vi "UMLEditor Main.vi"(1 "StartProject":string, 3 "StartTarget":string) -> ()   [LabVIEW 2012] (continued)
                                tunnel: w1808 -> [w1870 _ _ _]
                                tunnel: w1799 -> [w1869 _ _ _]
                                tunnel: w1806 -> [_ _ _ _]
                                tunnel: w1798 -> [w1868 _ _ _]
                                frame 0 {
                                n622 = case shown="False" w1870 {
                                tunnel: w1869 -> [_ _]
                                tunnel: w1868 -> [_ w1874]
                                frame False {
                                }
                                frame True {
                                n623 = call <resource>:"GDSProject_GetProjects.vi"("OpenProjectRef(True)"=FALSE) -> ("Projects"=w1877:string[], "error out"=w1880:errorcluster)  [unwired: 2 in, 15 out]
                                n624 = Array Size(array=w1877) -> (size(s)=w1876:i32)
                                n625 = Empty Array?(array=w1877) -> (empty?=w1881:bool)
                                n626 = Decrement(x=w1876) -> (x-1=w1875:i32)
                                n627 = Max & Min(x=w1875, y=w1874) -> (min(x,y)=w1873:i32)  [unwired: 1 out]
                                n628 = Max & Min(x=w1873, y=0) -> (max(x,y)=w1871:i32)  [unwired: 1 out]
                                n629 = Index Array(array=w1877, index=w1871) -> (element=w1879:string)
                                n630 = property on="Project" class="Ring (strict)"("Strings []"=w1877, "Value"=w1871) -> ()  [unwired: 2 in, 2 out]
                                n631 = case shown="False" w1881 {
                                tunnel: w1879 -> [w1887 _]
                                tunnel: w1880 -> [w1888 w1898]
                                tunnel: [w1885 w1897] -> _
                                frame False {
                                n632 = call <resource>:"GetRelativePathOption.vi"() -> ("UseProjectFolderAsBasePath"=w1890:bool)  [unwired: 1 in, 18 out]
                                n633 = call <resource>:"UMLEditor_TargetDialog.vi"("error in (no error)"=w1888, "Target"="My Computer" ("element"), "GetProjectRefByName"=w1887) -> ("error out"=w1885:errorcluster, "ProjectFolder"=w1886:path, "TargetIndex"=w1883:u16, "Targets"=w1884:string[])  [unwired: 4 in, 1 out]
                                n634 = case shown="True" w1890 {
                                tunnel: w1886 -> [_ w1892]
                                tunnel: File_StoredPathesActions."Set Path" ("Method (Get Path)") -> [_ w1891]
                                frame False {
                                }
                                frame True {
                                n635 = call <resource>:"File_ApplicationPaths.vi"("PathName"=UMLEditor_StoredPathes."ClassBasePath" ("UMLPathes"), "Path In"=w1892, "Method (Get Path)"=w1891) -> ()  [unwired: 1 in, 16 out]
                                }
                                }
                                n636 = property on="Target" class="Ring (strict)"("Strings []"=w1884, "Value"=w1883) -> ()  [unwired: 2 in, 2 out]
                                }
                                frame True {
                                n637 = call <resource>:"CommonVIs_UmlOpenVIRef.vi"("ProjectNameIn"="clear", "error in"=w1898) -> ("error out"=w1897:errorcluster)  [unwired: 2 in, 7 out]
                                n638 = property on="Target" class="Ring (strict)"("Strings []"=string[] [], "Value"=u16 0 ("icon")) -> ()  [unwired: 2 in, 2 out]
                                }
                                }
                                }
                                }
                                }
                                frame 1 {
                                }
                                frame 2 {
                                }
                                frame Default {
                                }
                                }
                                n639 = case shown="False" w1812 {
                                tunnel: w1814 -> [w1864 w1867]
                                tunnel: [w1864 w1866] -> w1813
                                frame False {
                                }
                                frame True {
                                n640 = Bundle By Name(cluster=w1867, "state"=UMLEditor_statesType."AddNodeFromProjectTree") -> (w1866:T7)
                                }
                                }
                              }
                              frame True {
                                n641 = Unbundle By Name(w1908) -> ("Cursors"=w1911:refnum<k1>[])
                                n642 = case shown="\"Expand\", \"Collaps\"" w1905 {
                                tunnel: w1911 -> [w1917 _]
                                tunnel: w1910 -> [w1913 w1923]
                                tunnel: [w1913 w1923] -> w1909
                                tunnel: w1905 -> [w1915 _]
                                tunnel: w1903 -> [w1912 w1922]
                                frame Default {
                                n643 = case shown="\"N\", \"S\"" w1915 {
                                tunnel: [_ UMLEditor_Cursortype."NS" ("CursorType") UMLEditor_Cursortype."NESW" ("CursorType") UMLEditor_Cursortype."WE" ("CursorType") UMLEditor_Cursortype."NWSE" ("CursorType")] -> w1914
                                frame Default {
                                }
                                frame "N", "S" {
                                }
                                frame "NE", "SW" {
                                }
                                frame "E", "W" {
                                }
                                frame "SE", "NW" {
                                }
                                }
                                n644 = Index Array(array=w1917, index=w1914) -> (element=w1916:refnum<k1>)
                                n645 = call-poly <vilib>:"Set Cursor.vi"("error in (no error)"=w1913, "VI reference (current VI)"=w1912, "cursor ID"=w1916) -> ()  [unwired: 9 out]
                                }
                                frame "Expand", "Collaps" {
                                n646 = call-poly <vilib>:"Set Cursor.vi"("error in (no error)"=w1923, "VI reference (current VI)"=w1922, "icon"=u16 6) -> ()  [unwired: 9 out]
                                }
                                }
                                n647 = Bundle By Name(cluster=w1907, "HotSpotNode"=w1904) -> (w1906:T7)
                              }
                            }
                          }
                          frame True {
                            n648 = property class="VI"() -> ("Front Panel.IsFrontmost"=w1926:bool)  [unwired: 2 in, 2 out]
                            n649 = case shown="True" w1926 {
                              tunnel: w1925 -> [_ w1945]
                              tunnel: w1934 -> [_ w1944]
                              tunnel: w1933 -> [_ w1943]
                              tunnel: w1932 -> [w1936 w1942]
                              tunnel: [w1936 w1941] -> w1931
                              tunnel: [w1935 w1940] -> w1930
                              tunnel: w1929 -> [w1935 w1939]
                              tunnel: w1928 -> [_ w1938]
                              tunnel: w1927 -> [_ w1937]
                              frame False {
                              }
                              frame True {
                                n650 = case shown="True" w1943 {
                                tunnel: w1945 -> [w1946 w1981]
                                tunnel: w1944 -> [w1974 _]
                                tunnel: w1942 -> [w1956 w1984]
                                tunnel: [w1956 w1985] -> w1941
                                tunnel: [w1968 w1983] -> w1940
                                tunnel: w1939 -> [w1968 w1982]
                                tunnel: w1938 -> [w1952 _]
                                tunnel: w1937 -> [_ _]
                                frame False {
                                w1960 = 0 ("lower limit")
                                n651 = Unbundle By Name(w1956) -> ("zoom"=w1953:dbl)
                                n652 = Multiply(x=w1953, y=w1974) -> (x*y=w1955:dbl)
                                n653 = Multiply(x=w1953, y=w1952) -> (x*y=w1954:dbl)
                                n654 = In Range and Coerce(upper limit=10, x=w1946, lower limit=-10) -> ()  [unwired: 2 out]
                                n655 = property on="Picture" class="Pict"() -> ("Draw Area Size"=w1977:T43)  [unwired: 2 in, 2 out]
                                n656 = To Long Integer(number=w1954) -> (32bit integer=w1964:i32)
                                n657 = To Long Integer(number=w1955) -> (32bit integer=w1971:i32)
                                n658 = property on="Picture" class="Pict"() -> ("Origin:Top"=w1950:i16, "Origin:Left"=w1959:i16)  [unwired: 2 in, 2 out]
                                n659 = Unbundle By Name(w1977) -> ("Height"=w1973:u32, "Width"=w1965:u32)
                                n660 = Subtract(x=w1950, y=w1946) -> (x-y=w1976:i32)
                                n661 = Subtract(x=w1959, y=w1946) -> (x-y=w1958:i32)
                                n662 = To Long Integer(number=w1965) -> (32bit integer=w1963:i32)
                                n663 = Subtract(x=w1964, y=w1963) -> (x-y=w1962:i32)
                                n664 = Max & Min(x=w1962, y=w1960) -> (max(x,y)=w1961:i32)  [unwired: 1 out]
                                n665 = In Range and Coerce(upper limit=w1961, x=w1958, lower limit=w1960) -> (coerced(x)=w1957:i32)  [unwired: 1 out]
                                n666 = To Long Integer(number=w1973) -> (32bit integer=w1966:i32)
                                n667 = Subtract(x=w1971, y=w1966) -> (x-y=w1972:i32)
                                n668 = Max & Min(x=w1972, y=0 ("lower limit")) -> (max(x,y)=w1969:i32)  [unwired: 1 out]
                                n669 = In Range and Coerce(upper limit=w1969, x=w1976, lower limit=0) -> (coerced(x)=w1951:i32)  [unwired: 1 out]
                                n670 = Not Equal?(x=w1951, y=w1950) -> (x != y?=w1949:bool)
                                n671 = Select(t=w1959, s=w1949, f=w1957) -> (s? t:f=w1967:i32)
                                n672 = property on="Picture" class="Pict"("Origin:Top"=w1951, "Origin:Left"=w1967) -> ()  [unwired: 2 in, 2 out]
                                }
                                frame True {
                                w1986 = 1.5 ("x")
                                n673 = Unbundle By Name(w1984) -> ("graphics"=w1993:refnum<class "Graphics.lvclass">, "zoom"=w1979:dbl)
                                n674 = Less Than 0?(x=w1981) -> (x < 0?=w1991:bool)
                                n675 = Not(x=w1991) -> (.not. x?=w1978:bool)
                                n676 = Multiply(x=w1979, y=w1986) -> (x*y=w1992:dbl)
                                n677 = Divide(x=w1979, y=w1986) -> (x/y=w1990:dbl)
                                n678 = Select(t=w1992, s=w1978, f=w1990) -> (s? t:f=w1989:dbl)
                                n679 = In Range and Coerce(upper limit=5.0625, x=w1989, lower limit=0.197530864) -> (coerced(x)=w1980:dbl)  [unwired: 1 out]
                                n680 = call <resource>:"scale.vi"("reference"=w1993, "scaleX"=w1980, "scaleY"=w1980, "error in (no error)"=w1982) -> ("error out"=w1983:errorcluster)  [unwired: 15 out]
                                n681 = Bundle By Name(cluster=w1984, "zoom"=w1980, "state"=UMLEditor_statesType."Repaint") -> (w1985:T7)
                                }
                                }
                              }
                            }
                          }
                        }
                        n682 = Bundle By Name(cluster=w1756, "HotSpotCursor"=w1754, "HotSpotFunction"=w1753) -> (w1755:T7)
                      }
                      frame True {
                        n683 = disable-structure shown="Disabled" {
                          frame Disabled {
                            n684 = property class="VI"() -> ("Front Panel Window:Panel Bounds"=w2011:T53)  [unwired: 2 in, 2 out]
                            n685 = Unbundle By Name(w2011) -> ("Left"=w2005:i16, "Top"=w2002:i16, "Right"=w2006:i16, "Bottom"=w2003:i16)
                            n686 = Subtract(x=w2003, y=w2002) -> (x-y=w2001:i16)
                            n687 = Subtract(x=w2006, y=w2005) -> (x-y=w2004:i16)
                            n688 = Subtract(x=w2004, y=23 ("X")) -> (x-y=w2010:i32)
                            n689 = Subtract(x=w2001, y=100) -> (x-y=w2009:i32)
                            n690 = Bundle(w2010, w2009) -> (w2000:cluster{i32, i32})  [unwired: 1 in]
                            n691 = property on="Picture" class="Pict"("Draw Area Size"=w2000) -> ()  [unwired: 2 in, 2 out]
                          }
                          frame Enabled {
                          }
                        }
                        n692 = Bundle By Name(cluster=w1999, "state"=UMLEditor_statesType."Repaint", "ResizePanelInProgress"=FALSE) -> (w1997:T7)
                      }
                    }
                  }
                  frame True {
                    n693 = property on="Picture" class="Pict"() -> ("Mouse"=w2016:T42)  [unwired: 2 in, 2 out]
                    n694 = Unbundle By Name(w2016) -> ("Mouse Position"=w2015:cluster{"X":i32, "Y":i32})
                    n695 = Unbundle By Name(w2014) -> ("zoom"=w2023:dbl, "offset"=w2021:T12)
                    n696 = Add(x=w2021, y=w2015) -> (x+y=w2022:T12)
                    n697 = Divide(x=w2022, y=w2023) -> (x/y=w2019:T12)
                    n698 = call-dynamic "findNode.vi"("reference"=w2012, "point2D"=w2019, "error in (no error)"=w2013) -> ("node"=w2020:refnum<class "AbstractNode.lvclass">, "found"=w2017:bool, "error out"=w2018:errorcluster)  [unwired: 13 in, 1 out]
                    n699 = case shown="True" w2017 {
                      tunnel: [w2025 w2028] -> w2024
                      tunnel: w2020 -> [_ w2032]
                      tunnel: w2019 -> [_ w2031]
                      tunnel: w2018 -> [w2025 w2030]
                      frame False {
                      }
                      frame True {
                        n700 = call-dynamic "GetContextHelpInfo.vi"("reference"=w2032, "MousePos"=w2031, "error in (no error)"=w2030) -> ("ContextHelpInfoExist"=w2026:bool, "ContextHelpInfo"=w2027:variant, "error out"=w2029:errorcluster)  [unwired: 13 in, 1 out]
                        n701 = case shown="True" w2026 {
                          tunnel: w2029 -> [w2033 w2036]
                          tunnel: [w2033 w2035] -> w2028
                          tunnel: w2027 -> [_ w2034]
                          frame False {
                          }
                          frame True {
                            n702 = call <resource>:"ContextHelp_SendMessageToPopUp.vi"("PopUpMessage"=w2034, "error in (no error)"=w2036) -> ("error out"=w2035:errorcluster)  [unwired: 1 in, 16 out]
                          }
                        }
                      }
                    }
                  }
                }
              }
              frame True {
                (unwired) UMLEditor_HotSpotType."Expand" ("HotSpotFunction")
                n703 = property on="Picture" class="Pict"() -> ("Mouse"=w2040:T42)  [unwired: 2 in, 2 out]
                n704 = Unbundle By Name(w2040) -> ("Mouse Position.X"=w2069:i32, "Mouse Position.Y"=w2068:i32, "Mouse Position"=w2051:cluster{"X":i32, "Y":i32})
                n705 = Unbundle By Name(w2039) -> ("graphics"=w2065:refnum<class "Graphics.lvclass">, "rubberBandStart"=w2064:T12, "dragStartPoint"=w2048:T12, "dragStartBounds"=w2056:T13, "selcted"=w2047:T9, "lastMousePoint"=w2046:T12)
                n706 = Unbundle By Name(w2039) -> ("HotSpotCursor"=w2042:bool, "HotSpotFunction"=w2044:T19)
                n707 = Unbundle By Name(w2039) -> ("ShiftDown"=w2038:bool, "CtrlDown"=w2037:bool)
                n708 = Unbundle By Name(w2039) -> ("selcted"=w2058:T9, "SelectedNodes"=w2057:refnum<class "AbstractNode.lvclass">[], "selectedEdge"=w2049:refnum<class "AbstractEdge.lvclass">)
                n709 = Unbundle By Name(w2039) -> ("offset"=w2050:T12, "zoom"=w2061:dbl)
                n710 = Add(x=w2051, y=w2050) -> (x+y=w2052:T12)
                n711 = Add(x=w2069, y=w2068) -> (x+y=w2067:i32)
                n712 = Divide(x=w2052, y=w2061) -> (x/y=w2053:T12)
                n713 = Equal?(x=w2046, y=w2053) -> (x = y?=w2054:bool)
                n714 = call <resource>:"Point getValues.vi"("point2D"=w2064) -> ("valid"=w2063:bool)  [unwired: 18 out]
                n715 = call <resource>:"Point getValues.vi"("point2D"=w2048) -> ("valid"=w2062:bool)  [unwired: 18 out]
                n716 = Less Than 0?(x=w2067) -> (x < 0?=w2055:bool)
                n717 = Or(x=w2054, y=w2055) -> (x .or. y?=w2043:bool)
                n718 = Compound Arithmetic op=AND(w2043, invert w2042) -> (w2041:bool)
                n719 = case shown="True" w2041 {
                  tunnel: w2053 -> [w2091 _]
                  tunnel: w2065 -> [w2090 _]
                  tunnel: w2039 -> [w2078 w2314]
                  tunnel: [w2077 w2313] -> w2066
                  tunnel: w2064 -> [w2089 _]
                  tunnel: w2063 -> [w2088 _]
                  tunnel: w2062 -> [w2087 _]
                  tunnel: w2059 -> [w2086 w2312]
                  tunnel: [w2085 w2312] -> w2060
                  tunnel: w2039 -> [w2084 _]
                  tunnel: w2058 -> [w2083 _]
                  tunnel: w2057 -> [w2082 _]
                  tunnel: w2056 -> [w2081 _]
                  tunnel: w2048 -> [w2080 _]
                  tunnel: w2045 -> [w2079 _]
                  tunnel: w2054 -> [_ w2311]
                  tunnel: w2049 -> [w2076 _]
                  tunnel: w2047 -> [w2075 _]
                  tunnel: w2046 -> [w2074 _]
                  tunnel: w2045 -> [w2073 _]
                  tunnel: w2042 -> [w2072 _]
                  tunnel: w2044 -> [w2071 _]
                  tunnel: w2038 -> [_ _]
                  tunnel: w2037 -> [_ _]
                  tunnel: w2037 -> [w2070 _]
                  frame False {
                    n720 = case shown="False" w2088 {
                      tunnel: w2091 -> [w2102 w2279]
                      tunnel: w2090 -> [_ w2286]
                      tunnel: w2089 -> [_ w2280]
                      tunnel: w2087 -> [w2109 _]
                      tunnel: w2086 -> [w2107 w2285]
                      tunnel: [w2108 w2284] -> w2085
                      tunnel: w2084 -> [w2106 _]
                      tunnel: w2083 -> [w2105 _]
                      tunnel: w2082 -> [w2104 _]
                      tunnel: w2081 -> [w2103 _]
                      tunnel: w2080 -> [w2101 _]
                      tunnel: w2079 -> [w2100 _]
                      tunnel: w2078 -> [w2099 w2283]
                      tunnel: [w2098 w2282] -> w2077
                      tunnel: w2076 -> [w2097 _]
                      tunnel: w2075 -> [_ w2281]
                      tunnel: w2074 -> [w2096 _]
                      tunnel: w2073 -> [w2095 _]
                      tunnel: w2072 -> [w2094 _]
                      tunnel: w2071 -> [w2093 _]
                      tunnel: w2070 -> [w2092 _]
                      frame False {
                        n721 = case shown="True" w2109 {
                          tunnel: [w2111 w2125] -> w2108
                          tunnel: w2107 -> [w2111 w2126]
                          tunnel: w2106 -> [_ _]
                          tunnel: w2105 -> [_ w2127]
                          tunnel: w2104 -> [_ w2124]
                          tunnel: w2103 -> [_ w2117]
                          tunnel: w2102 -> [_ w2123]
                          tunnel: w2101 -> [_ w2122]
                          tunnel: w2100 -> [_ w2121]
                          tunnel: w2099 -> [w2110 w2120]
                          tunnel: [w2110 w2119] -> w2098
                          tunnel: w2097 -> [_ w2118]
                          tunnel: w2096 -> [_ w2116]
                          tunnel: w2095 -> [_ w2115]
                          tunnel: w2094 -> [_ w2114]
                          tunnel: w2093 -> [_ w2113]
                          tunnel: w2092 -> [_ w2112]
                          frame False {
                          }
                          frame True {
                            n722 = case shown="\"Edge\"" w2127 {
                              tunnel: w2126 -> [w2129 w2136 w2256]
                              tunnel: [w2129 w2140 w2264] -> w2125
                              tunnel: w2124 -> [_ w2134 w2255]
                              tunnel: w2123 -> [_ w2137 w2254]
                              tunnel: w2122 -> [_ _ w2270]
                              tunnel: w2121 -> [_ _ w2267]
                              tunnel: w2120 -> [w2128 w2142 w2266]
                              tunnel: [w2128 w2138 w2262] -> w2119
                              tunnel: w2118 -> [_ _ w2261]
                              tunnel: w2117 -> [_ _ _]
                              tunnel: w2116 -> [_ w2135 _]
                              tunnel: w2115 -> [_ w2133 _]
                              tunnel: w2114 -> [_ w2132 _]
                              tunnel: w2113 -> [_ w2131 _]
                              tunnel: w2112 -> [_ w2130 _]
                              frame Default {
                              }
                              frame "Node" {
                                n723 = Bundle By Name(cluster=w2142, "state"=UMLEditor_statesType."Repaint", "lastMousePoint"=w2137) -> (w2139:T7)
                                n724 = case shown="True" w2132 {
                                tunnel: [w2150 w2206] -> w2140
                                tunnel: w2139 -> [w2149 w2202]
                                tunnel: [w2148 w2201] -> w2138
                                tunnel: w2137 -> [w2147 w2210]
                                tunnel: w2136 -> [w2146 w2207]
                                tunnel: w2135 -> [w2145 w2209]
                                tunnel: w2134 -> [w2144 w2205]
                                tunnel: w2133 -> [_ _]
                                tunnel: w2131 -> [_ w2208]
                                tunnel: w2130 -> [w2143 _]
                                frame False {
                                n725 = case shown="False" w2143 {
                                tunnel: [w2160 w2196] -> w2150
                                tunnel: w2149 -> [w2159 w2200]
                                tunnel: [w2158 w2197] -> w2148
                                tunnel: w2147 -> [w2157 _]
                                tunnel: w2146 -> [w2156 w2196]
                                tunnel: w2145 -> [w2155 _]
                                tunnel: w2144 -> [w2154 _]
                                frame False {
                                n726 = for {
                                tunnel: w2154 -> [w2163] mode=indexing
                                shift-right: [w2164] -> w2153
                                shift-left: refnum<class "AbstractNode.lvclass">[] [] -> [w2165]
                                n727 = call <resource>:"GetAllChildrenRecursive.vi"("reference"=w2163) -> ("children"=w2162:refnum<class "AbstractNode.lvclass">[])  [unwired: 1 in, 17 out]
                                n728 = Build Array (concatenate)(w2165, w2162) -> (w2164:refnum<class "AbstractNode.lvclass">[])
                                }
                                n729 = for {
                                tunnel: w2154 -> [w2189] mode=indexing
                                tunnel: w2157 -> [w2185]
                                shift-right: [w2187] -> w2152
                                shift-left: w2156 -> [w2188]
                                tunnel: w2155 -> [w2184]
                                tunnel: w2153 -> [w2171]
                                w2174 = 0.0 ("t")
                                n730 = Subtract(x=w2185, y=w2184) -> (x-y=w2186:T12)
                                n731 = call-dynamic "getBounds.vi"("reference"=w2189, "error in (no error)"=w2188) -> ("reference out"=w2168:refnum<class "AbstractNode.lvclass">, "bounds"=w2183:T13, "error out"=w2169:errorcluster)  [unwired: 15 in]
                                n732 = Unbundle(w2183) -> ("x"=w2182:dbl, "y"=w2176:dbl)  [unwired: 2 out]
                                n733 = Unbundle(w2186) -> ("x"=w2175:dbl, "y"=w2173:dbl)
                                n734 = call-dynamic "getParent.vi"("reference"=w2168, "error in (no error)"=w2169) -> ("reference out"=w2166:refnum<class "AbstractNode.lvclass">, "error out"=w2167:errorcluster)  [unwired: 13 in, 3 out]
                                n735 = Search 1D Array(1D array=w2171, element=w2168) -> (index of element=w2170:i32)  [unwired: 1 out]
                                n736 = Add(x=w2182, y=w2175) -> (x+y=w2181:dbl)
                                n737 = Add(x=w2176, y=w2173) -> (x+y=w2177:dbl)
                                n738 = Less Than 0?(x=w2181) -> (x < 0?=w2180:bool)
                                n739 = Less Than 0?(x=w2177) -> (x < 0?=w2178:bool)
                                n740 = Select(t=w2174, s=w2180, f=w2175) -> (s? t:f=w2179:dbl)
                                n741 = Select(t=w2174, s=w2178, f=w2173) -> (s? t:f=w2172:dbl)
                                n742 = case shown="-1" w2170 {
                                tunnel: w2167 -> [w2190 w2195]
                                tunnel: [w2190 w2194] -> w2187
                                tunnel: w2179 -> [_ w2193]
                                tunnel: w2172 -> [_ w2192]
                                tunnel: w2166 -> [_ w2191]
                                frame 0, Default {
                                }
                                frame -1 {
                                n743 = call-dynamic "translate.vi"("reference"=w2191, "dx"=w2193, "dy"=w2192, "error in (no error)"=w2195) -> ("error out"=w2194:errorcluster)  [unwired: 14 in, 1 out]
                                }
                                }
                                }
                                n744 = call <resource>:"UMLEditor setDiagramInfo.vi"("error in (no error)"=w2152, "localVariablesIn"=w2159, "action"=enum16{"Name/Dir", "Unsaved", "Saved"}."Unsaved") -> ("localVariablesOut"=w2158:T7, "error out"=w2160:errorcluster)  [unwired: 2 in, 13 out]
                                }
                                frame True {
                                n745 = Bundle By Name(cluster=w2200, "state"=UMLEditor_statesType."CopyPaste", "CtrlDown"=FALSE) -> (w2197:T7)
                                }
                                }
                                }
                                frame True {
                                n746 = Subtract(x=w2210, y=w2209) -> (x-y=w2211:T12)
                                n747 = Unbundle(w2211) -> ("x"=w2204:dbl, "y"=w2203:dbl)
                                n748 = case shown="\"Expand\", \"Collaps\"" w2208 {
                                selector: w2208 -> [_ w2219 w2236]
                                tunnel: w2207 -> [w2213 w2218 w2241]
                                tunnel: [w2213 w2216 w2240] -> w2206
                                tunnel: w2205 -> [_ w2217 w2239]
                                tunnel: w2204 -> [_ _ w2238]
                                tunnel: w2203 -> [_ _ w2237]
                                tunnel: w2202 -> [w2212 w2215 w2235]
                                tunnel: [w2212 w2214 w2235] -> w2201
                                frame Default {
                                }
                                frame "Expand", "Collaps" {
                                n749 = disable-structure shown="Disabled" {
                                disable-tunnel: w2219 -> [w2232 _]
                                disable-tunnel: w2218 -> [w2229 w2233]
                                disable-tunnel: w2217 -> [w2228 _]
                                disable-tunnel: [w2224 w2233] -> w2216
                                disable-tunnel: w2215 -> [w2223 w2234]
                                disable-tunnel: [w2220 w2234] -> w2214
                                frame Disabled {
                                n750 = Index Array(array=w2228) -> (element=w2227:refnum<class "AbstractNode.lvclass">)  [unwired: 1 in]
                                n751 = Equal?(x=w2232, y=UMLEditor_HotSpotType."Collaps") -> (x = y?=w2230:bool)
                                n752 = call-dynamic "Collaps.vi"("reference in"=w2227, "Collaps"=w2230, "error in (no error)"=w2229) -> ("error out"=w2225:errorcluster)  [unwired: 15 in, 1 out]
                                n753 = Bundle By Name(cluster=w2223, "HotSpotCursor"=FALSE) -> (w2221:T7)
                                n754 = call <resource>:"UMLEditor setDiagramInfo.vi"("error in (no error)"=w2225, "localVariablesIn"=w2221, "action"=enum16{"Name/Dir", "Unsaved", "Saved"}."Unsaved") -> ("localVariablesOut"=w2220:T7, "error out"=w2224:errorcluster)  [unwired: 2 in, 13 out]
                                }
                                frame Enabled {
                                }
                                }
                                }
                                frame "N".."NW" {
                                n755 = for {
                                shift-right: [w2246] -> w2240
                                shift-left: w2241 -> [w2247]
                                tunnel: w2239 -> [w2245] mode=indexing
                                tunnel: w2238 -> [w2244]
                                tunnel: w2237 -> [w2243]
                                tunnel: w2236 -> [w2242]
                                n756 = call-dynamic "Resize.vi"("reference in"=w2245, "dx"=w2244, "dy"=w2243, "Positions"=w2242, "error in (no error)"=w2247) -> ("error out"=w2246:errorcluster)  [unwired: 13 in, 1 out]
                                }
                                }
                                }
                                }
                                }
                              }
                              frame "Edge" {
                                n757 = Array Size(array=w2255) -> (size(s)=w2248:i32)
                                n758 = Unbundle By Name(w2270) -> ("x"=w2269:dbl, "y"=w2268:dbl)
                                n759 = case shown="2" w2248 {
                                tunnel: w2255 -> [_ w2274]
                                tunnel: [w2272 w2273] -> w2250
                                frame 2 {
                                n760 = call <resource>:"GetObject.vi"("RefNum"=-1 ("type")) -> ("reference"=w2272:refnum<class "AbstractNode.lvclass">)  [unwired: 17 in, 1 out]
                                }
                                frame Default {
                                n761 = Index Array(array=w2274) -> (element=w2273:refnum<class "AbstractNode.lvclass">)  [unwired: 1 in]
                                }
                                }
                                n762 = Unbundle(w2254) -> ("x"=w2258:dbl, "y"=w2257:dbl)
                                n763 = Subtract(x=w2258, y=w2269) -> (x-y=w2260:dbl)
                                n764 = Subtract(x=w2257, y=w2268) -> (x-y=w2259:dbl)
                                n765 = Bundle By Name(cluster=w2266, "state"=UMLEditor_statesType."Repaint", "lastMousePoint"=w2254, "dragStartPoint"=w2254) -> (w2263:T7)
                                n766 = call-dynamic "Translate.vi"("reference"=w2261, "dx"=w2260, "dy"=w2259, "StartEndNode"=w2250, "error in (no error)"=w2256) -> ("error out"=w2251:errorcluster)  [unwired: 13 in, 1 out]
                                n767 = case shown="False" "Case Constant\n(See Context Help) 2" {
                                tunnel: w2267 -> [_ w2278]
                                tunnel: [w2275 w2277] -> w2252
                                tunnel: w2251 -> [w2275 w2276]
                                frame False {
                                }
                                frame True {
                                n768 = call-dynamic "layout.vi"("reference"=w2278, "error in (no error)"=w2276) -> ("error out"=w2277:errorcluster)  [unwired: 16 in, 1 out]
                                }
                                }
                                n769 = call <resource>:"UMLEditor setDiagramInfo.vi"("error in (no error)"=w2252, "localVariablesIn"=w2263, "action"=enum16{"Name/Dir", "Unsaved", "Saved"}."Unsaved") -> ("localVariablesOut"=w2262:T7, "error out"=w2264:errorcluster)  [unwired: 2 in, 13 out]
                              }
                            }
                          }
                        }
                      }
                      frame True {
                        n770 = case shown="\"None\"" w2281 {
                          tunnel: w2286 -> [w2302 w2310]
                          tunnel: w2285 -> [w2304 w2309]
                          tunnel: [w2303 w2308] -> w2284
                          tunnel: w2280 -> [w2297 w2306]
                          tunnel: w2279 -> [w2296 w2305]
                          frame "None" {
                            n771 = Unbundle(w2297) -> ("x"=w2295:dbl, "y"=w2291:dbl)
                            n772 = Unbundle(w2296) -> ("x"=w2294:dbl, "y"=w2290:dbl)
                            n773 = Max & Min(x=w2295, y=w2294) -> (max(x,y)=w2293:dbl, min(x,y)=w2292:dbl)
                            n774 = Max & Min(x=w2291, y=w2290) -> (max(x,y)=w2289:dbl, min(x,y)=w2288:dbl)
                            n775 = Subtract(x=w2293, y=w2292) -> (x-y=w2299:dbl)
                            n776 = Subtract(x=w2289, y=w2288) -> (x-y=w2298:dbl)
                            n777 = Bundle By Name(cluster=T13 {"x"=0.0, "y"=0.0, "width"=0.0, "height"=0.0} ("rectangle"), "x"=w2292, "y"=w2288, "width"=w2299, "height"=w2298) -> (w2287:T13)
                            n778 = call <resource>:"drawTempRectangle.vi"("reference"=w2302, "rectangle"=w2287, "color(if not used=default color)"=u32 16711680, "error in (no error)"=w2304) -> ("error out"=w2303:errorcluster)  [unwired: 4 in, 11 out]
                          }
                          frame Default {
                            n779 = Build Array(w2306, w2305) -> (w2307:T12[])
                            n780 = call-dynamic "drawTempLine.vi"("reference"=w2310, "points"=w2307, "error in (no error)"=w2309) -> ("error out"=w2308:errorcluster)  [unwired: 15 in, 1 out]
                          }
                        }
                        n781 = Bundle By Name(cluster=w2283, "lastMousePoint"=w2279) -> (w2282:T7)
                      }
                    }
                  }
                  frame True {
                    n782 = case shown="True" w2311 {
                      tunnel: w2314 -> [w2318 w2320]
                      tunnel: [w2317 w2320] -> w2313
                      frame False {
                        w2316 = T12 {"x"=nan, "y"=nan} ("rubberBandStart")
                        n783 = Bundle By Name(cluster=w2318, "butDwn"=FALSE ("b_dwn"), "rubberBandStart"=w2316, "dragStartPoint"=w2316, "dragStartBounds"=T13 {"x"=nan, "y"=nan, "width"=nan, "height"=nan}) -> (w2317:T7)
                      }
                      frame True {
                      }
                    }
                  }
                }
              }
            }
          }
          event User Event {
            # "WholeProject"
            # "ReverseEngineering:Class:%s:%s"
            n784 = event-data() -> ("Action"=w2322:string, "Data"=w2321:string)  [unwired: 1 out]
            n785 = case shown="\"ReverseEngineering\"" w2322 {
              tunnel: w2326 -> [w2328 w2352 w2405 w2426]
              tunnel: [w2328 w2351 w2404 w2425] -> w2325
              tunnel: w2321 -> [_ w2350 w2403 w2427]
              tunnel: w2324 -> [w2327 w2348 w2401 w2423]
              tunnel: [w2327 w2347 w2400 w2423] -> w2323
              frame "False", Default {
              }
              frame "ReverseEngineering" {
                n786 = Match Pattern(string=w2350, regular expression=":") -> (before substring=w2337:string, after substring=w2345:string)  [unwired: 3 out]
                n787 = Match Pattern(string=w2345, regular expression=":") -> (before substring=w2344:string, after substring=w2335:string)  [unwired: 3 out]
                n788 = Reverse String(1:w2335) -> (0:w2334:string)
                n789 = Match Pattern(string=w2334, regular expression=":") -> (before substring=w2333:string, after substring=w2332:string)  [unwired: 3 out]
                n790 = Reverse String(1:w2333) -> (0:w2330:string)
                n791 = Reverse String(1:w2332) -> (0:w2331:string)
                n792 = call <resource>:"GDSProject_GetProjects.vi"("error in (no error)"=w2348, "OpenProjectRef(True)"=FALSE) -> ("Projects"=w2340:string[], "error out"=w2342:errorcluster)  [unwired: 1 in, 15 out]
                n793 = case shown="\"WholeProject\"" w2337 {
                  tunnel: w2352 -> [w2356 w2360 w2364]
                  tunnel: [w2355 w2359 w2363] -> w2351
                  tunnel: w2337 -> [w2354 _ _]
                  tunnel: w2331 -> [_ w2357 w2361]
                  frame "WholeProject" {
                    n794 = Bundle By Name(cluster=w2356, "Action"=w2354, "state"=UMLEditor_statesType."ClassReversedEngineering") -> (w2355:T7)
                  }
                  frame Default {
                    n795 = Bundle By Name(cluster=w2360, "Action"=w2357, "state"=UMLEditor_statesType."ClassReversedEngineering") -> (w2359:T7)
                  }
                  frame "VI" {
                    n796 = Bundle By Name(cluster=w2364, "Action"=w2361, "state"=UMLEditor_statesType."AddNodeFromProjectTree+SyncAll") -> (w2363:T7)
                  }
                }
                n797 = Search 1D Array(1D array=w2340, element=w2344) -> (index of element=w2339:i32)  [unwired: 1 out]
                n798 = case shown="0, Default" w2339 {
                  selector: w2339 -> [w2365 _]
                  tunnel: [w2365 0 ("t")] -> w2338
                  frame 0, Default {
                  }
                  frame -1 {
                  }
                }
                n799 = Index Array(array=w2340, index=w2338) -> (element=w2343:string)
                n800 = Empty Array?(array=w2340) -> (empty?=w2341:bool)
                n801 = property on="Project" class="Ring (strict)"("Strings []"=w2340, "Value"=w2338) -> ()  [unwired: 2 in, 2 out]
                n802 = case shown="True" w2341 {
                  tunnel: w2343 -> [w2374 _]
                  tunnel: w2342 -> [w2375 w2381]
                  tunnel: [w2373 w2381] -> w2347
                  tunnel: w2330 -> [w2370 _]
                  frame False {
                    n803 = call <resource>:"UMLEditor_TargetDialog.vi"("error in (no error)"=w2375, "Target"=w2370, "GetProjectRefByName"=w2374) -> ("error out"=w2373:errorcluster, "ProjectFolder"=w2367:path, "TargetIndex"=w2371:u16, "Targets"=w2372:string[])  [unwired: 4 in, 1 out]
                    n804 = call <resource>:"GetRelativePathOption.vi"() -> ("UseProjectFolderAsBasePath"=w2369:bool)  [unwired: 1 in, 18 out]
                    n805 = case shown="True" w2369 {
                      tunnel: w2367 -> [_ w2377]
                      tunnel: File_StoredPathesActions."Set Path" ("Method (Get Path)") -> [_ w2376]
                      frame False {
                      }
                      frame True {
                        n806 = call <resource>:"File_ApplicationPaths.vi"("PathName"=UMLEditor_StoredPathes."ClassBasePath" ("UMLPathes"), "Path In"=w2377, "Method (Get Path)"=w2376) -> ()  [unwired: 1 in, 16 out]
                      }
                    }
                    n807 = property on="Target" class="Ring (strict)"("Strings []"=w2372, "Value"=w2371) -> ()  [unwired: 2 in, 2 out]
                  }
                  frame True {
                    n808 = property on="Target" class="Ring (strict)"("Strings []"=string[] [], "Value"=u16 0 ("icon")) -> ()  [unwired: 2 in, 2 out]
                  }
                }
              }
              frame "ShowInStateDiagram" {
                n809 = Match Pattern(string=w2403, regular expression=":") -> (after substring=w2398:string)  [unwired: 4 out]
                n810 = Match Pattern(string=w2398, regular expression=":") -> (before substring=w2397:string, after substring=w2383:string)  [unwired: 3 out]
                n811 = Reverse String(1:w2383) -> (0:w2388:string)
                n812 = Match Pattern(string=w2388, regular expression=":") -> (before substring=w2387:string, after substring=w2386:string)  [unwired: 3 out]
                n813 = Reverse String(1:w2387) -> (0:w2384:string)
                n814 = Reverse String(1:w2386) -> (0:w2385:string)
                n815 = call <resource>:"GDSProject_GetProjects.vi"("error in (no error)"=w2401, "OpenProjectRef(True)"=FALSE) -> ("Projects"=w2393:string[], "error out"=w2395:errorcluster)  [unwired: 1 in, 15 out]
                n816 = Search 1D Array(1D array=w2393, element=w2397) -> (index of element=w2392:i32)  [unwired: 1 out]
                n817 = case shown="-1" w2392 {
                  selector: w2392 -> [w2406 _]
                  tunnel: [w2406 0 ("t")] -> w2391
                  frame 0, Default {
                  }
                  frame -1 {
                  }
                }
                n818 = Index Array(array=w2393, index=w2391) -> (element=w2396:string)
                n819 = Empty Array?(array=w2393) -> (empty?=w2394:bool)
                n820 = property on="Project" class="Ring (strict)"("Strings []"=w2393, "Value"=w2391) -> ()  [unwired: 2 in, 2 out]
                n821 = case shown="True" w2394 {
                  tunnel: w2396 -> [w2415 _]
                  tunnel: w2395 -> [w2416 w2422]
                  tunnel: [w2414 w2422] -> w2400
                  tunnel: w2384 -> [w2411 _]
                  frame False {
                    n822 = call <resource>:"UMLEditor_TargetDialog.vi"("error in (no error)"=w2416, "Target"=w2411, "GetProjectRefByName"=w2415) -> ("error out"=w2414:errorcluster, "ProjectFolder"=w2408:path, "TargetIndex"=w2412:u16, "Targets"=w2413:string[])  [unwired: 4 in, 1 out]
                    n823 = call <resource>:"GetRelativePathOption.vi"() -> ("UseProjectFolderAsBasePath"=w2410:bool)  [unwired: 1 in, 18 out]
                    n824 = property on="Target" class="Ring (strict)"("Strings []"=w2413, "Value"=w2412) -> ()  [unwired: 2 in, 2 out]
                    n825 = case shown="True" w2410 {
                      tunnel: w2408 -> [_ w2418]
                      tunnel: File_StoredPathesActions."Set Path" ("Method (Get Path)") -> [_ w2417]
                      frame False {
                      }
                      frame True {
                        n826 = call <resource>:"File_ApplicationPaths.vi"("PathName"=UMLEditor_StoredPathes."ClassBasePath" ("UMLPathes"), "Path In"=w2418, "Method (Get Path)"=w2417) -> ()  [unwired: 1 in, 16 out]
                      }
                    }
                  }
                  frame True {
                    n827 = property on="Target" class="Ring (strict)"("Strings []"=string[] [], "Value"=u16 0 ("icon")) -> ()  [unwired: 2 in, 2 out]
                  }
                }
                n828 = Bundle By Name(cluster=w2405, "Action"=w2385, "state"=UMLEditor_statesType."AnalyseViInStateDiagram") -> (w2404:T7)
              }
              frame "OpenUmlFile" {
                n829 = String To Path(string=w2427) -> (path=w2424:path)
                n830 = Bundle By Name(cluster=w2426, "state"=UMLEditor_statesType."Open", "file"=w2424) -> (w2425:T7)
              }
            }
          }
          event Key Down?; event type 5.0.x8000000b {
            (unwired) eventvkey."ASCII" ("VKey")
            n831 = event-data() -> ("Type"=w2434:T55, "Char"=w2442:i16, "VKey"=w2432:T54, "PlatMods"=w2441:T56)  [unwired: 3 out]
            n832 = Unbundle By Name(w2430) -> ("SelectedNodes"=w2436:refnum<class "AbstractNode.lvclass">[], "graphics"=w2433:refnum<class "Graphics.lvclass">)
            n833 = disable-structure shown="Disabled" {
              disable-tunnel: w2430 -> [w2445 w2447]
              disable-tunnel: [w2444 w2447] -> w2429
              frame Disabled {
                w2446 = FALSE ("Sync")
                n834 = Bundle By Name(cluster=w2445, "Sync"=w2446) -> (w2444:T7)
                n835 = local write "Sync"(w2446) -> ()
              }
              frame Enabled {
              }
            }
            n836 = Unbundle By Name(w2441) -> ("Ctrl"=w2431:bool, "Shift"=w2435:bool)
            n837 = case shown="\"Shift\"" w2432 {
              tunnel: w2432 -> [w2458 _ _ _]
              tunnel: w2429 -> [w2457 w2629 w2711 w2714]
              tunnel: [w2456 w2629 w2710 w2714] -> w2443
              tunnel: w2442 -> [w2455 _ _ _]
              tunnel: [w2453 w2628 w2709 w2713] -> w2440
              tunnel: w2439 -> [w2454 w2627 w2709 w2713]
              tunnel: w2438 -> [w2451 w2626 _ _]
              tunnel: w2430 -> [w2450 w2625 _ _]
              tunnel: w2437 -> [_ w2624 _ _]
              tunnel: w2436 -> [w2452 _ _ _]
              tunnel: w2435 -> [w2449 _ _ _]
              tunnel: w2434 -> [_ w2623 _ _]
              tunnel: w2433 -> [_ w2622 _ _]
              tunnel: w2431 -> [w2448 _ _ _]
              frame Default {
                n838 = case shown="False" w2448 {
                  tunnel: w2458 -> [w2468 _]
                  tunnel: w2457 -> [w2467 w2620]
                  tunnel: [w2466 w2620] -> w2456
                  tunnel: w2455 -> [w2465 _]
                  tunnel: w2454 -> [w2464 w2621]
                  tunnel: [w2463 w2621] -> w2453
                  tunnel: w2452 -> [w2462 _]
                  tunnel: w2451 -> [w2461 _]
                  tunnel: w2450 -> [w2460 _]
                  tunnel: w2449 -> [w2459 _]
                  frame False {
                    n839 = case shown="\"ASCII\"" w2468 {
                      selector: w2468 -> [_ _ _ w2549 _]
                      tunnel: w2467 -> [w2483 w2532 w2538 w2551 w2619]
                      tunnel: [w2486 w2531 w2537 w2552 w2619] -> w2466
                      tunnel: w2465 -> [w2481 _ _ _ _]
                      tunnel: w2464 -> [w2475 w2530 w2535 w2557 w2618]
                      tunnel: [w2474 w2530 w2535 w2556 w2618] -> w2463
                      tunnel: w2462 -> [_ _ _ w2555 _]
                      tunnel: w2461 -> [w2473 _ _ w2553 _]
                      tunnel: w2460 -> [_ _ _ w2550 _]
                      tunnel: w2459 -> [_ _ _ w2546 _]
                      frame "ASCII" {
                        n840 = Build Array(w2481) -> (w2480:i16[])
                        n841 = local read "SearchString"() -> (w2479:string)
                        n842 = Byte Array To String(unsigned byte array=w2480) -> (string=w2478:string)
                        n843 = Concatenate Strings(w2479, w2478) -> (w2472:string)
                        "SearchString" <- w2472
                        n844 = call <vilib>:"Trim Whitespace.vi"("string"=w2472) -> ("trimmed string"=w2477:string)  [unwired: 1 in]
                        n845 = Match Pattern(string=w2472, regular expression="^!") -> (after substring=w2469:string, offset past match=w2470:i32)  [unwired: 1 in, 2 out]
                        n846 = Equal?(x=w2481, y=i16 32) -> (x = y?=w2485:bool)
                        n847 = String Length(string=w2477) -> (length=w2476:i32)
                        n848 = Tick Count (ms)() -> (millisecond timer value=w2482:u32)
                        n849 = Bundle By Name(cluster=w2483, "KeyPressTime"=w2482) -> (w2484:T7)
                        n850 = case shown="0" w2476 {
                          tunnel: [w2495 w2524] -> w2486
                          tunnel: w2485 -> [_ w2523]
                          tunnel: w2484 -> [w2494 w2522]
                          tunnel: w2475 -> [w2493 w2521]
                          tunnel: [w2492 w2521] -> w2474
                          tunnel: w2472 -> [w2491 _]
                          tunnel: w2473 -> [w2490 _]
                          tunnel: w2470 -> [w2489 _]
                          tunnel: w2469 -> [w2488 _]
                          frame Default {
                            n851 = case shown="-1" w2489 {
                              tunnel: [w2498 w2512] -> w2495
                              tunnel: w2494 -> [w2498 w2511]
                              tunnel: w2493 -> [w2497 w2510]
                              tunnel: [w2497 w2509] -> w2492
                              tunnel: w2491 -> [_ w2508]
                              tunnel: w2490 -> [_ w2507]
                              tunnel: w2488 -> [w2500 _]
                              frame 0, Default {
                                n852 = Match Pattern(string=w2500, regular expression="!$") -> (before substring=w2496:string, offset past match=w2499:i32)  [unwired: 1 in, 2 out]
                                n853 = case shown="0, Default" w2499 {
                                tunnel: w2496 -> [w2502 _]
                                frame 0, Default {
                                n854 = property on="PictureMenuEvent" class="Str"("Val(Sgnl)"=w2502) -> ()  [unwired: 2 in, 2 out]
                                n855 = local write "SearchString"("" ("SearchString")) -> ()
                                }
                                frame -1 {
                                }
                                }
                              }
                              frame -1 {
                                n856 = call-dynamic "FindNodeByName.vi"("reference"=w2507, "Name"=w2508, "error in (no error)"=w2510) -> ("node"=w2506:refnum<class "AbstractNode.lvclass">, "found"=w2505:bool, "error out"=w2509:errorcluster)  [unwired: 13 in, 1 out]
                                n857 = case shown="True" w2505 {
                                tunnel: [w2513 w2517] -> w2512
                                tunnel: w2511 -> [w2513 w2516]
                                tunnel: w2506 -> [_ w2515]
                                frame False {
                                }
                                frame True {
                                n858 = Build Array(w2515) -> (w2518:refnum<class "AbstractNode.lvclass">[])
                                n859 = Bundle By Name(cluster=w2516, "state"=UMLEditor_statesType."PanAndRepaint", "selcted"=UMLEditor_tooltype."Node", "SelectedNodes"=w2518, "newSelected"=TRUE) -> (w2517:T7)
                                }
                                }
                                n860 = property on="SearchString" class="Str"("Visible"=TRUE) -> ()  [unwired: 2 in, 2 out]
                              }
                            }
                          }
                          frame 0 {
                            n861 = case shown="True" w2523 {
                              tunnel: [w2525 w2529] -> w2524
                              tunnel: w2522 -> [w2525 w2528]
                              frame False {
                              }
                              frame True {
                                n862 = call <resource>:"UMLEditor UpdatesToolbuttons.vi"() -> ()  [unwired: 6 in, 14 out]
                                n863 = Bundle By Name(cluster=w2528, "toolType"=UMLEditor_tooltype."None", "tool"=UMLEditor_toolsType."CD_Select") -> (w2529:T7)
                              }
                            }
                          }
                        }
                      }
                      frame "Enter", "Return" {
                        n864 = Bundle By Name(cluster=w2532, "state"=UMLEditor_statesType."EditSelected") -> (w2531:T7)
                      }
                      frame "Delete" {
                        n865 = Bundle By Name(cluster=w2538, "state"=UMLEditor_statesType."RemoveSelected", "Don'tDeleteChildren"=FALSE) -> (w2537:T7)
                      }
                      frame "Up".."Right" {
                        w2554 = refnum<class "AbstractNode.lvclass">[] []
                        n866 = Unbundle By Name(w2550) -> ("gridSize"=w2544:dbl)
                        n867 = Select(t=5.0, s=w2546, f=1.0 ("t")) -> (s? t:f=w2545:dbl)
                        n868 = for {
                          tunnel: w2555 -> [w2580] mode=indexing
                          shift-right: [w2581] -> w2560
                          shift-left: w2554 -> [w2582]
                          n869 = call <resource>:"GetAllChildrenRecursive.vi"("reference"=w2580) -> ("children"=w2579:refnum<class "AbstractNode.lvclass">[])  [unwired: 1 in, 17 out]
                          n870 = Build Array (concatenate)(w2582, w2579) -> (w2581:refnum<class "AbstractNode.lvclass">[])
                        }
                        n871 = Multiply(x=w2545, y=w2544) -> (x*y=w2543:dbl)
                        n872 = case shown="\"Left\"" w2549 {
                          tunnel: w2543 -> [w2566 w2567 w2570 w2572]
                          tunnel: [0.0 ("t") 0.0 ("t") w2569 w2572] -> w2548
                          tunnel: [w2564 w2567 0.0 ("t") 0.0 ("t")] -> w2547
                          frame "Up" {
                            n873 = Negate(x=w2566) -> (-x=w2564:dbl)
                          }
                          frame "Down" {
                          }
                          frame "Left" {
                            n874 = Negate(x=w2570) -> (-x=w2569:dbl)
                          }
                          frame "Right", Default {
                          }
                        }
                        n875 = for {
                          tunnel: w2555 -> [w2607] mode=indexing
                          shift-right: [w2605] -> w2559
                          shift-left: w2557 -> [w2606]
                          tunnel: w2560 -> [w2594]
                          shift-right: [w2587] -> w2540
                          shift-left: w2554 -> [w2588]
                          tunnel: w2548 -> [w2585]
                          tunnel: w2547 -> [w2584]
                          w2596 = 0.0 ("t")
                          n876 = call-dynamic "getBounds.vi"("reference"=w2607, "error in (no error)"=w2606) -> ("reference out"=w2591:refnum<class "AbstractNode.lvclass">, "bounds"=w2604:T13, "error out"=w2592:errorcluster)  [unwired: 15 in]
                          n877 = Unbundle(w2604) -> ("x"=w2603:dbl, "y"=w2597:dbl)  [unwired: 2 out]
                          n878 = call-dynamic "getParent.vi"("reference"=w2591, "error in (no error)"=w2592) -> ("reference out"=w2589:refnum<class "AbstractNode.lvclass">, "parentNode"=w2586:refnum<class "AbstractNode.lvclass">, "ValidParent"=w2583:bool, "error out"=w2590:errorcluster)  [unwired: 13 in, 1 out]
                          n879 = Search 1D Array(1D array=w2594, element=w2591) -> (index of element=w2593:i32)  [unwired: 1 out]
                          n880 = Add(x=w2603, y=w2585) -> (x+y=w2602:dbl)
                          n881 = Add(x=w2597, y=w2584) -> (x+y=w2598:dbl)
                          n882 = Less Than 0?(x=w2602) -> (x < 0?=w2601:bool)
                          n883 = Less Than 0?(x=w2598) -> (x < 0?=w2599:bool)
                          n884 = case shown="True" w2583 {
                            tunnel: w2588 -> [w2608 w2611]
                            tunnel: [w2608 w2610] -> w2587
                            tunnel: w2586 -> [_ w2609]
                            frame False {
                            }
                            frame True {
                              n885 = Build Array (concatenate)(w2611, w2609) -> (w2610:refnum<class "AbstractNode.lvclass">[])
                            }
                          }
                          n886 = Select(t=w2596, s=w2601, f=w2585) -> (s? t:f=w2600:dbl)
                          n887 = Select(t=w2596, s=w2599, f=w2584) -> (s? t:f=w2595:dbl)
                          n888 = case shown="-1" w2593 {
                            tunnel: w2590 -> [w2612 w2617]
                            tunnel: [w2612 w2616] -> w2605
                            tunnel: w2600 -> [_ w2615]
                            tunnel: w2595 -> [_ w2614]
                            tunnel: w2589 -> [_ w2613]
                            frame 0, Default {
                            }
                            frame -1 {
